vi "Tooling-Root.vi"(8 "error in (no error)":errorcluster) -> (0 "error out":errorcluster, 3 "Root":path)   [LabVIEW 2018, in "Scripting.lvlib"]
uses:
  Scripting.lvlib
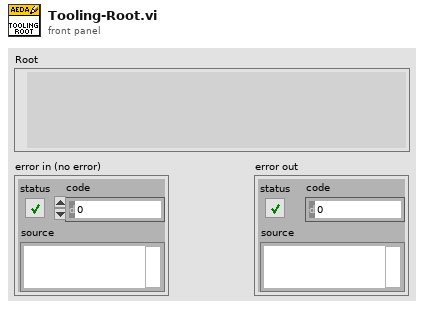
[diagram p1: front panel]
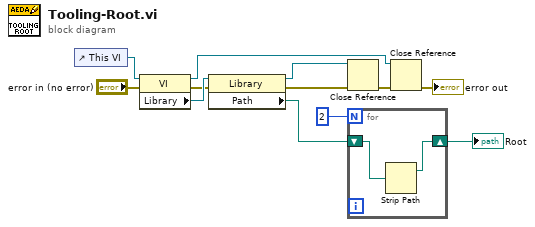
[diagram p0: block diagram]
diagram:
  n1 = control-ref of="This VI"() -> (w12:refnum<vi>)
  n2 = property class="VI"(reference=w12, error in="error in (no error)") -> (reference out=w5:refnum<vi>, error out=w10:errorcluster, "Library"=w11:refnum<vi>)
  n3 = property class="Library"(reference=w11, error in=w10) -> (reference out=w7:refnum<vi>, error out=w8:errorcluster, "Path"=w9:path)
  n4 = Close Reference(reference=w7, error in (no error)=w8) -> (error out=w6:errorcluster)
  n5 = for {
    N: 2 -> [_]
    shift-right: [w13] -> w2
    shift-left: w9 -> [w14]
    n6 = Strip Path(path=w14) -> (stripped path=w13:path)  [unwired: 1 out]
  }
  "Root" <- w2
  n7 = Close Reference(reference=w5, error in (no error)=w6) -> (error out=→"error out":errorcluster)
